vi "CommandDynamixelPositionNoNotifiers.vi"(6 "Mode control":T2=enum."RC_control", 7 "Dynamixel Bounds":T4={"Main Dynamixel Set Data"={"Lower Winch Bound (deg)"=0.0, "Upper Winch Bound (deg)"=800.0}, "Rudder Dynamixel Set Data"={"Lower Winch Bound (deg)"=0.0, "Upper Winch Bound (deg)"=30.0}, "Jib Dynamixel Set Data"={"Lower Winch Bound (deg)"=0.0, "Upper Winch Bound (deg)"=800.0}}, 8 "error in":errorcluster, 9 "FPGA VI Reference In":refnum<k20>, 10 "Dynamixel Cycles":T3, 11 "VISA resource name":refnum<visa-resource-name>) -> (0 "Error out":errorcluster, 2 "Commanded rudder value":T1 min=-0.95 max=0.95 scale=1.0..-1.0, 3 "Commanded sail value":dbl)   [LabVIEW 2013]
doc: "First thing to know is that there is a Control Mode switch in this VI that you can switch between RC testing and hand testing.\n\nWhen RC testing, this VI checks the FPGA for RC data, bounds it so that the data is from 0-1 in steps of 0.05, converts that 0-1 value (or -1 to 1 for the rudder) into Dynamixel degrees (1200 dynamixel counts per 360 degrees) and then writes that position to the Dynamixel. This is highly dependent on the motor bounds which are passed in from above, because a sail value of 1 means different things when the motor bounds are different.\n\nHand test has the same process for commanding the motors but the input method is a control.\n\nEric Schneider, October 2014"
uses:
  Data/TypeDefs/Rudder Set Suggestions.ctl
  Data/TypeDefs/Sail Set Suggestions.ctl
  Data/TypeDefs/MotorSetup.ctl
  Data/TypeDefs/DynamixelSetupInfo.ctl
  Data/TypeDefs/DynamixelCycleTracker.ctl
  Data/TypeDefs/HindbrainControlOptions.ctl
  <vilib>/rvi/interface/common/niFpgaWaitOnOcc.vi
  <vilib>/Utility/error.llb/Error Cluster From Error Code.vi
  <vilib>/rvi/errors/niLvFpgaAdjustHostInterfaceError.vi
  <vilib>/rvi/interface/nirviReadWriteControl/nirviReadWriteControl.xnode
  NiFpgaLv.dll
  <vilib>/rvi/interface/Simulation/niFpgaSimulationCallBeginRW.vi
panel:
  out "Rudder written value":dbl
  out "Main written value":dbl
  in  "Hand Sail Control":T6 {"MainSailSuggestion" min=0.0 max=1.0; "JibSailSuggestion" min=0.0 max=1.0}
  in  "Suggested Rudder Setpoint":T1 min=-0.95 max=0.95 scale=1.0..-1.0
  out "Jib written value":dbl
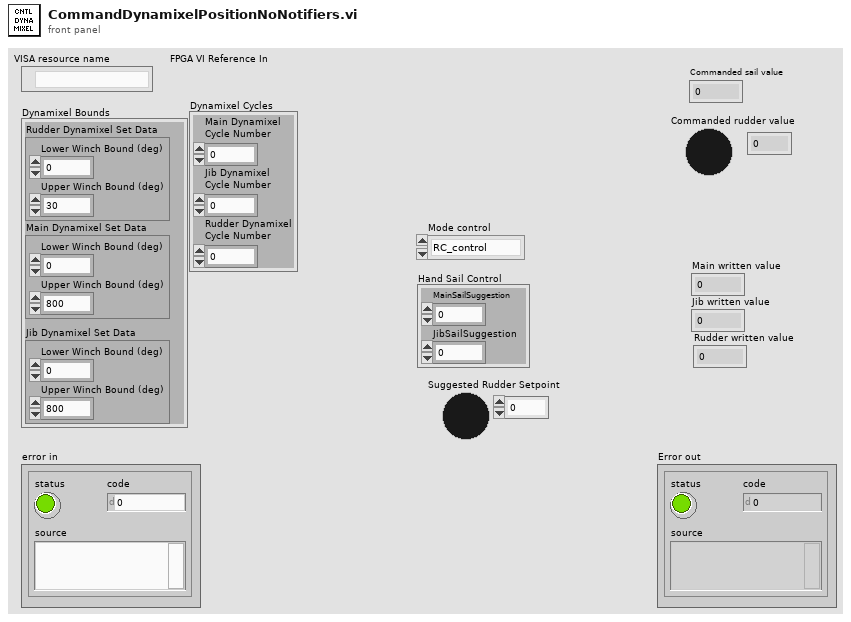
[diagram p1: front panel]
types:
  T1 = typedef "Rudder Set Suggestions.ctl" = dbl
  T2 = typedef "HindbrainControlOptions.ctl" = enum16{"code_control", "RC_control", "hand_control"}
  T3 = typedef "DynamixelCycleTracker.ctl" = cluster{"Main Dynamixel\nCycle Number":i32, "Jib Dynamixel\nCycle Number":i32, "Rudder Dynamixel\nCycle Number":i32}
  T4 = typedef "MotorSetup.ctl" = cluster{"Main Dynamixel Set Data":T5, "Rudder Dynamixel Set Data":T5, "Jib Dynamixel Set Data":T5}
  T5 = typedef "DynamixelSetupInfo.ctl" = cluster{"Lower Winch Bound (deg)":dbl, "Upper Winch Bound (deg)":dbl}
  T6 = typedef "Sail Set Suggestions.ctl" = cluster{"MainSailSuggestion":dbl, "JibSailSuggestion":dbl}
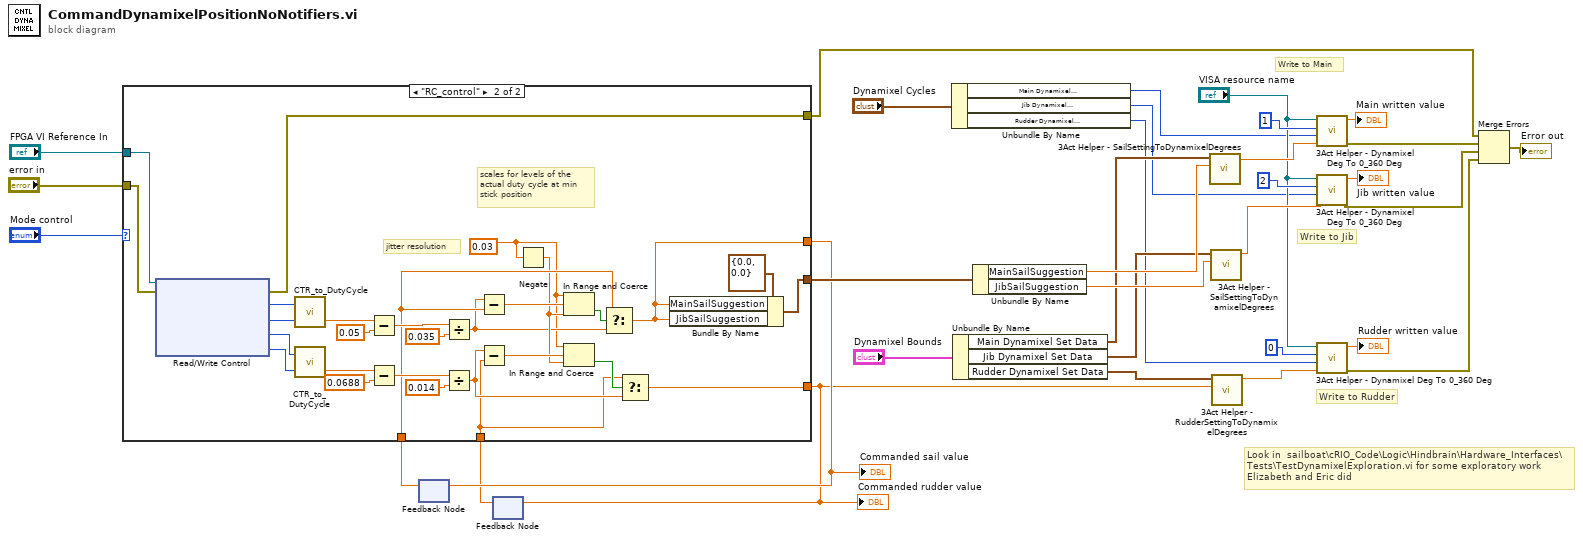
[diagram p0: block diagram]
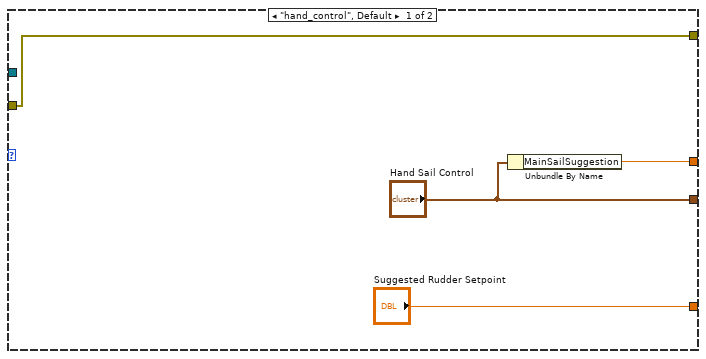
[diagram p2: hidden frame]
diagram:
  # "Look in  sailboat\\cRIO_Code\\Logic\\Hindbrain\\Hardware_Interfaces\\Tests\\TestDynamixelExploration.vi for some exploratory work Elizabeth and Eric did"
  # "Write to Rudder"
  # "Write to Jib"
  # "Write to Main"
  n1 = feedback #1() -> (w5:dbl)  [unwired: 1 in]
  n2 = feedback #2() -> (w3:T1)  [unwired: 1 in]
  n3 = case shown="\"RC_control\"" "Mode control" {
    tunnel: ["Suggested Rudder Setpoint" w43] -> w4
    tunnel: ["Hand Sail Control" w64] -> w13
    tunnel: "FPGA VI Reference In" -> [_ w61]
    tunnel: "error in" -> [w36 w52]
    tunnel: [w36 w51] -> w7
    tunnel: [w34 w42] -> w6
    tunnel: w5 -> [_ w48]
    tunnel: w3 -> [_ w44]
    frame "hand_control", Default {
      n4 = Unbundle By Name("Hand Sail Control") -> ("MainSailSuggestion"=w34:dbl)
    }
    frame "RC_control" {
      w38 = 0.03 ("Jitter cutout")
      # "jitter resolution"
      # "scales for levels of the\nactual duty cycle at min\nstick position"
      n5 = xnode "Read/Write Control"("FPGA VI Reference In"=w61, "error in"=w52) -> ("error out"=w51:errorcluster, "Sail High Center"=w66:u32, "Sail Low Center"=w65:u32, "Rudder High Center"=w63:u32, "Rudder Low Center"=w62:u32)  [unwired: 1 out]
      n6 = call "CTR_to_DutyCycle.vi"("LOW CTR"=w65, "HIGH CTR"=w66) -> ("duty cycle fraction [0-1]"=w59:dbl)  [unwired: 1 out]
      n7 = call "CTR_to_DutyCycle.vi"("LOW CTR"=w62, "HIGH CTR"=w63) -> ("duty cycle fraction [0-1]"=w53:dbl)  [unwired: 1 out]
      n8 = Subtract(x=w59, y=0.05) -> (x-y=w58:dbl)
      n9 = Subtract(x=w53, y=0.0688) -> (x-y=w55:dbl)
      n10 = Divide(x=w58, y=0.035) -> (x/y=w39:dbl)
      n11 = Divide(x=w55, y=0.014) -> (x/y=w45:dbl)
      n12 = Subtract(x=w39, y=w48) -> (x-y=w50:dbl)
      n13 = Subtract(x=w45, y=w44) -> (x-y=w47:T1)
      n14 = Negate(x=w38) -> (-x=w40:dbl)
      n15 = In Range and Coerce(upper limit=w38, x=w50, lower limit=w40) -> (In Range?=w49:bool)  [unwired: 1 out]
      n16 = In Range and Coerce(upper limit=w38, x=w47, lower limit=w40) -> (In Range?=w46:bool)  [unwired: 1 out]
      n17 = Select(t=w48, s=w49, f=w39) -> (s? t:f=w42:dbl)
      n18 = Select(t=w44, s=w46, f=w45) -> (s? t:f=w43:T1)
      n19 = Bundle By Name(cluster=T6 {"MainSailSuggestion"=0.0, "JibSailSuggestion"=0.0} ("Hand Sail Control"), "MainSailSuggestion"=w42, "JibSailSuggestion"=w42) -> (w64:T6)
    }
  }
  "Commanded rudder value" <- w4
  "Commanded sail value" <- w6
  n20 = feedback-in #1(w6) -> ()
  n21 = feedback-in #2(w4) -> ()
  n22 = Unbundle By Name("Dynamixel Cycles") -> ("Main Dynamixel\nCycle Number"=w16:i32, "Jib Dynamixel\nCycle Number"=w15:i32, "Rudder Dynamixel\nCycle Number"=w14:i32)
  n23 = Unbundle By Name("Dynamixel Bounds") -> ("Main Dynamixel Set Data"=w23:T5, "Jib Dynamixel Set Data"=w18:T5, "Rudder Dynamixel Set Data"=w24:T5)
  n24 = Unbundle By Name(w13) -> ("MainSailSuggestion"=w33:dbl, "JibSailSuggestion"=w32:dbl)
  n25 = call "3Act Helper - SailSettingToDynamixelDegrees.vi"("SailSuggestion"=w33, "Dynamixel Set Data"=w23) -> ("Dynamixel Angle"=w28:dbl)  [unwired: 9 in]
  n26 = call "3Act Helper - SailSettingToDynamixelDegrees.vi"("SailSuggestion"=w32, "Dynamixel Set Data"=w18) -> ("Dynamixel Angle"=w27:dbl)  [unwired: 9 in]
  n27 = call "3Act Helper - RudderSettingToDynamixelDegrees.vi"("Suggested Rudder Setpoint"=w4, "Dynamixel Set Data"=w24) -> ("Dynamixel Angle"=w25:dbl)  [unwired: 9 in]
  n28 = call "3Act Helper - Dynamixel Deg To 0_360 Deg.vi"("Dynamixel Setpoint In (deg)"=w28, "Dynamixel Cycle Number"=w16, "Motor ID"=u8 1 ("Motor ID (0)"), "VISA resource name"="VISA resource name") -> ("Error out"=w22:errorcluster, "Written value"=→"Main written value":dbl)  [unwired: 6 in]
  n29 = call "3Act Helper - Dynamixel Deg To 0_360 Deg.vi"("Dynamixel Setpoint In (deg)"=w27, "Dynamixel Cycle Number"=w15, "Motor ID"=u8 2 ("Motor ID (0)"), "VISA resource name"="VISA resource name") -> ("Error out"=w21:errorcluster, "Written value"=→"Jib written value":dbl)  [unwired: 6 in]
  n30 = call "3Act Helper - Dynamixel Deg To 0_360 Deg.vi"("Dynamixel Setpoint In (deg)"=w25, "Dynamixel Cycle Number"=w14, "Motor ID"=u8 0 ("Motor ID (0)"), "VISA resource name"="VISA resource name") -> ("Error out"=w20:errorcluster, "Written value"=→"Rudder written value":dbl)  [unwired: 6 in]
  n31 = Merge Errors(w7, w22, w21, w20) -> (→"Error out":errorcluster)
